vi "ReadLowSetpoint.vi"(8 "error in (no error)":errorcluster, 11 "VISA resource name":refnum<visa-resource-name>) -> (0 "error out":errorcluster, 1 "LowChamberSetPoint":dbl, 2 "LowChamberSetPoint":string, 3 "VISA resource name out":refnum<visa-resource-name>)   [LabVIEW 2017, in "Thermal Shock.lvlib"]
uses:
  Thermal Shock.lvlib
  <vilib>/Instr/_visa.llb/VISA Configure Serial Port (Instr).vi
panel:
  in  "Read!":bool=TRUE
  out "Uncalculated Buffer":string
  in  "Stop":bool=TRUE
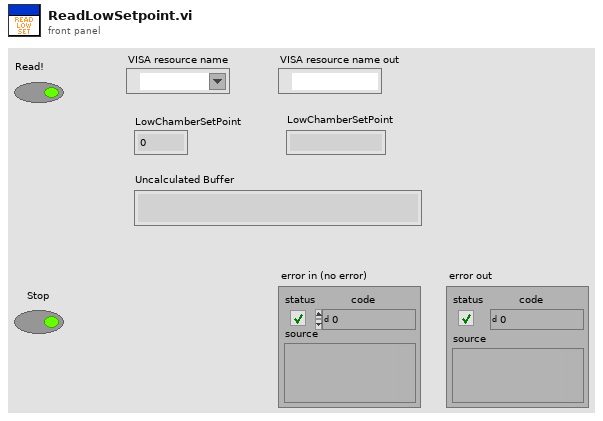
[diagram p1: front panel]
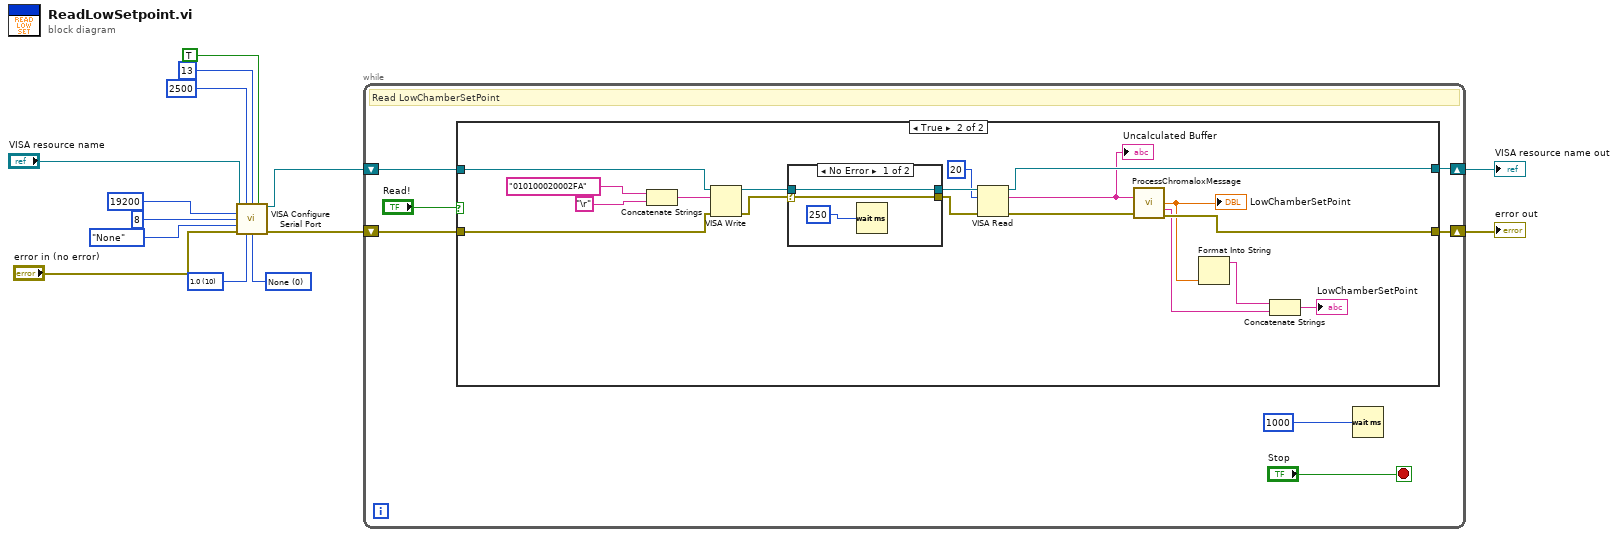
[diagram p0: block diagram]
diagram:
  w4 = u16 0 items=["None", "XON/XOFF", "RTS/CTS", "XON/XOFF & RTS/CTS", "DTR/DSR", "XON/XOFF & DTR/DSR"] ("flow control (0:none)")
  w6 = u16 10 items=["1.0"=10, "1.5"=15, "2.0"=20] ("stop bits (10: 1 bit)")
  n1 = call-poly "VISA Configure Serial Port"("VISA resource name"="VISA resource name", "timeout (10sec)"=2500, "termination char\n(0xA = '\\n' = LF)"=u8 13, "Enable Termination\nChar (T)"=TRUE, "baud rate (9600)"=19200, "data bits (8)"=u16 8, "parity (0:none)"=enum16{"None", "Odd", "Even", "Mark", "Space"}."None", "error in (no error)"="error in (no error)", "stop bits (10: 1 bit)"=w6, "flow control (0:none)"=w4) -> ("VISA resource name out"=w12:refnum<visa-resource-name>, "error out"=w14:errorcluster)  [unwired: 4 in]
  n2 = while {
    shift-right: [w16] -> w2
    shift-left: w12 -> [w19]
    shift-right: [w15] -> w1
    shift-left: w14 -> [w18]
    stop <- "Stop" stop-if-true
    # "Read LowChamberSetPoint"
    n3 = case shown="True" "Read!" {
      tunnel: w19 -> [w23 w31]
      tunnel: [w23 w33] -> w16
      tunnel: [w22 w29] -> w15
      tunnel: w18 -> [w22 w32]
      frame False {
      }
      frame True {
        n4 = Concatenate Strings("010100020002FA", "\r") -> (w39:string)
        n5 = VISA Write(VISA resource name=w31, write buffer=w39, error in (no error)=w32) -> (VISA resource name out=w36:refnum<visa-resource-name>, error out=w38:errorcluster)  [unwired: 1 out]
        n6 = case shown="No Error" w38 {
          selector: w38 -> [w44 w46]
          tunnel: [w44 w46] -> w37
          tunnel: w36 -> [w43 w45]
          tunnel: [w43 w45] -> w35
          frame No Error {
            n7 = Wait (ms)(milliseconds to wait=250) -> ()  [unwired: 1 out]
          }
          frame Error {
          }
        }
        n8 = VISA Read(VISA resource name=w35, byte count=20, error in (no error)=w37) -> (VISA resource name out=w33:refnum<visa-resource-name>, read buffer=w30:string, error out=w28:errorcluster)  [unwired: 1 out]
        "Uncalculated Buffer" <- w30
        n9 = call "ProcessChromaloxMessage.vi"("Chromalox Message"=w30, "error in (no error)"=w28) -> ("Reading"=w27:dbl, "Units"=w25:string, "error out"=w29:errorcluster)  [unwired: 10 in, 1 out]
        "LowChamberSetPoint" <- w27
        n10 = Format Into String(w27) -> (resulting string=w26:string)  [unwired: 3 in, 1 out]
        n11 = Concatenate Strings(w26, w25) -> (→"LowChamberSetPoint":string)
      }
    }
    n12 = Wait (ms)(milliseconds to wait=1000) -> ()  [unwired: 1 out]
  }
  "error out" <- w1
  "VISA resource name out" <- w2
